vi "Sound Player_.vi"() -> ()   [LabVIEW 2025]
doc: "This VI illustrates how to play a sound file directly to the speakers. It uses Play Sound File.vi which opens a file and starts playing immediately and asynchronously (as opposed to the method shown in Sound File to Sound Output.vi example)."
uses:
  <vilib>/sound2/lvsound2.llb/Sound Data Format.ctl
  <vilib>/sound2/lvsound2.llb/Sound Output Write (DBL).vi
panel:
  in  "Is output stereo?":bool=TRUE
  in  "Wet(K)":dbl(slide)=1.0 min=0.0 max=1.0 scale=0.0..1.0
  out "data in":waveform(dbl)[](graph)
  out "data out":waveform(dbl)[](graph)
  in  "Tail":i32=100000 min=0
  in  "Scale g":dbl=1.0 min=0.0
  in  "Scale N":dbl=2.0 min=0.0
  in  "path":path
  in  "Stop":bool
  in  "Device ID":u32
  out "Sound Is Playing?":bool
  # "Overview: Demonstrates the use of the Sound Functions to play a sound file.\nInstructions:\n1. Specify the Device ID.\n2. Run the VI. It may take a several seconds to load the file and start playing the sound."
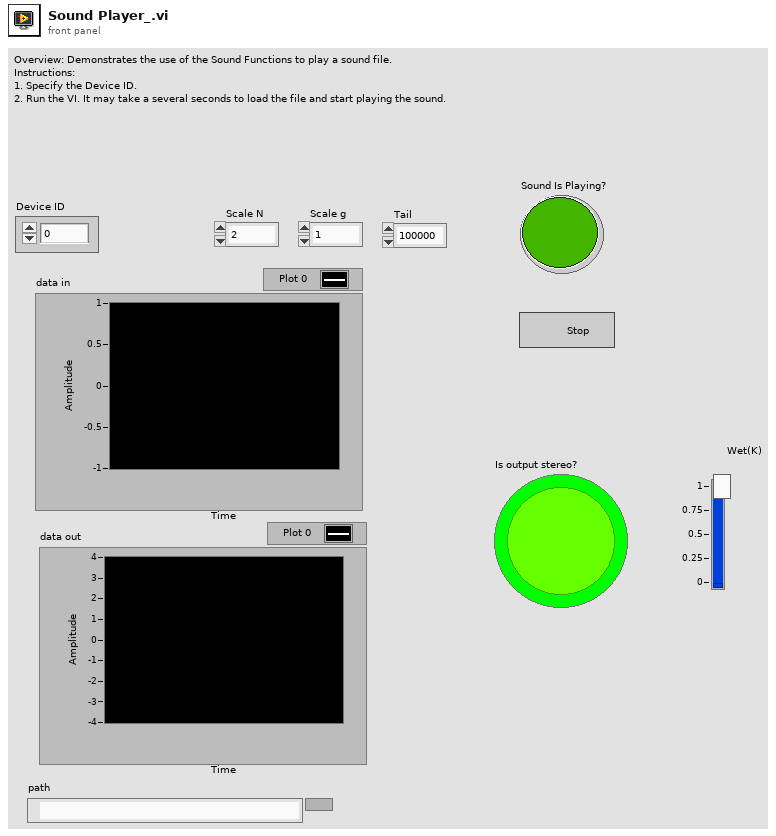
[diagram p1: front panel]
types:
  T1 = typedef "Sound Data Format.ctl" = cluster{"sample rate (S/s)":dbl, "number of channels":i32, "bits per sample":i32}
  T2 = typedef "Sound Output Task ID.ctl" = u32
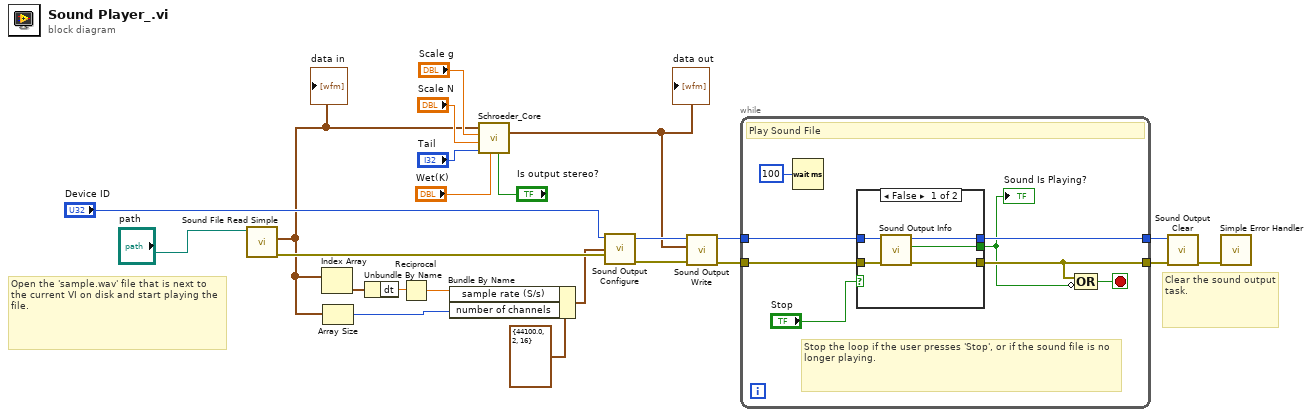
[diagram p0: block diagram]
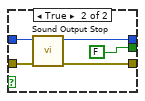
[diagram p2: hidden frame]
diagram:
  # "Clear the sound output task."
  # "Open the 'sample.wav' file that is next to the current VI on disk and start playing the file."
  n1 = call <vilib>:"Sound File Read Simple.vi"("path"="path") -> ("error out"=w19:errorcluster, "data"=w2:waveform(dbl)[])  [unwired: 7 in, 2 out]
  "data in" <- w2
  n2 = Index Array(array=w2) -> (element=w17:waveform(dbl))  [unwired: 1 in]
  n3 = Array Size(array=w2) -> (size(s)=w14:i32)
  n4 = Unbundle By Name(w17) -> ("dt"=w16:dbl)
  n5 = Reciprocal(x=w16) -> (1/x=w15:dbl)
  n6 = Bundle By Name(cluster=T1 {"sample rate (S/s)"=44100.0, "number of channels"=2, "bits per sample"=16} ("sound format"), "sample rate (S/s)"=w15, "number of channels"=w14) -> (w13:T1)
  n7 = call "Schroeder_Core.vi"("Is output stereo?"="Is output stereo?", "Wet(k)"="Wet(K)", "Tail"="Tail", "Scale N"="Scale N", "Scale g"="Scale g", "Data in (array)"=w2) -> ("Data out (array)"=w1:waveform(dbl)[])  [unwired: 5 in]
  "data out" <- w1
  n8 = call <vilib>:"Sound Output Configure.vi"("error in (no error)"=w19, "sound format"=w13, "device ID"="Device ID") -> ("error out"=w11:errorcluster, "task ID"=w10:T2)  [unwired: 7 in]
  n9 = call-poly <vilib>:"Sound Output Write.vi"("error in (no error)"=w11, "data"=w1, "task ID"=w10) -> ("error out"=w8:errorcluster, "task ID out"=w9:T2)  [unwired: 7 in]
  n10 = while {
    tunnel: w9 -> [w25]
    tunnel: [w30] -> w22
    tunnel: w8 -> [w26]
    tunnel: [w29] -> w23
    stop <- w31 stop-if-true
    # "Stop the loop if the user presses 'Stop', or if the sound file is no longer playing."
    # "Play Sound File"
    n11 = Wait (ms)(milliseconds to wait=u32 100) -> ()  [unwired: 1 out]
    n12 = case shown="False" "Stop" {
      tunnel: w26 -> [w36 w40]
      tunnel: [w35 w38] -> w30
      tunnel: w25 -> [w34 w41]
      tunnel: [w33 w39] -> w29
      tunnel: [w32 FALSE] -> w28
      frame False {
        n13 = call <vilib>:"Sound Output Info.vi"("error in (no error)"=w36, "task ID"=w34) -> ("error out"=w33:errorcluster, "is playing?"=w32:bool, "task ID out"=w35:T2)  [unwired: 6 in, 1 out]
      }
      frame True {
        n14 = call <vilib>:"Sound Output Stop.vi"("error in (no error)"=w40, "task ID"=w41) -> ("error out"=w39:errorcluster, "task ID out"=w38:T2)  [unwired: 8 in]
      }
    }
    "Sound Is Playing?" <- w28
    n15 = Compound Arithmetic op=OR(w29, invert w28) -> (w31:bool)
  }
  n16 = call <vilib>:"Sound Output Clear.vi"("error in (no error)"=w23, "task ID"=w22) -> ("error out"=w21:errorcluster)  [unwired: 9 in]
  n17 = call <vilib>:"Simple Error Handler.vi"("error in (no error)"=w21) -> ()  [unwired: 4 in, 5 out]
